vi "Time.vi"(1 "TestResult In":refnum<class "TestResult.lvclass">) -> (0 "Time":dbl)   [LabVIEW 2019, in "TestResult.lvclass"]
doc: "Returns the time for test execution (cumulative) in seconds."
uses:
  TestResult.lvclass
  TestResult.lvclass/TestResult.ctl
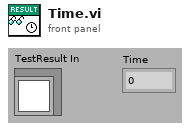
[diagram p1: front panel]
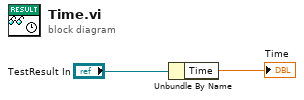
[diagram p0: block diagram]
diagram:
  n1 = Unbundle By Name("TestResult In") -> ("Time"=→"Time":dbl)
